vi "send_voltagePulse-v03.vi"(0 "daq_ao":tag="Dev1/ao1", 1 "daq_ai":tag="Dev1/ai0:1", 5 "VoltageRampValuesCluster":T2, 7 "Sample Freq (Hz)":dbl min=0.0 max=40000.0, 9 "set holding (mV)":dbl, 13 "Number of Replicates":i16=1 min=1 max=10, 14 "error in":errorcluster) -> (4 "output cluster":T1, 6 "output waveform":waveform(dbl)[](graph), 8 "protocol response":waveform(dbl)[](graph) caption="jumptestMonitor", 10 "error out":errorcluster)   [LabVIEW 2019]
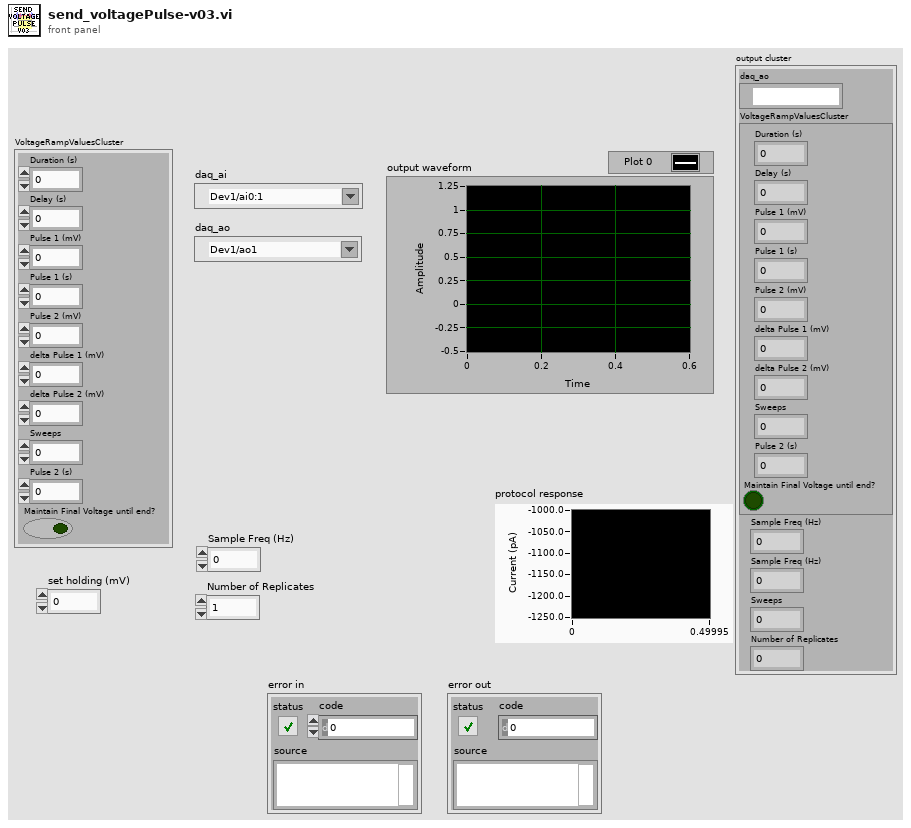
[diagram p1: front panel]
types:
  T1 = cluster{"daq_ao":tag, "VoltageRampValuesCluster":cluster{"Duration (s)":dbl, "Delay (s)":dbl, "Pulse 1 (mV)":dbl, "Pulse 1 (s)":dbl, "Pulse 2 (mV)":dbl, "delta Pulse 1 (mV)":dbl, "delta Pulse 2 (mV)":dbl, "Sweeps":dbl, "Pulse 2 (s)":dbl, "Maintain Final Voltage until end?":bool}, "Sample Freq (Hz)":dbl, "Sample Freq (Hz)":dbl, "Sweeps":dbl, "Number of Replicates":i16}
  T2 = cluster{"Duration (s)":dbl, "Delay (s)":dbl, "Pulse 1 (mV)":dbl, "Pulse 1 (s)":dbl, "Pulse 2 (mV)":dbl, "delta Pulse 1 (mV)":dbl, "delta Pulse 2 (mV)":dbl, "Sweeps":dbl, "Pulse 2 (s)":dbl, "Maintain Final Voltage until end?":bool}
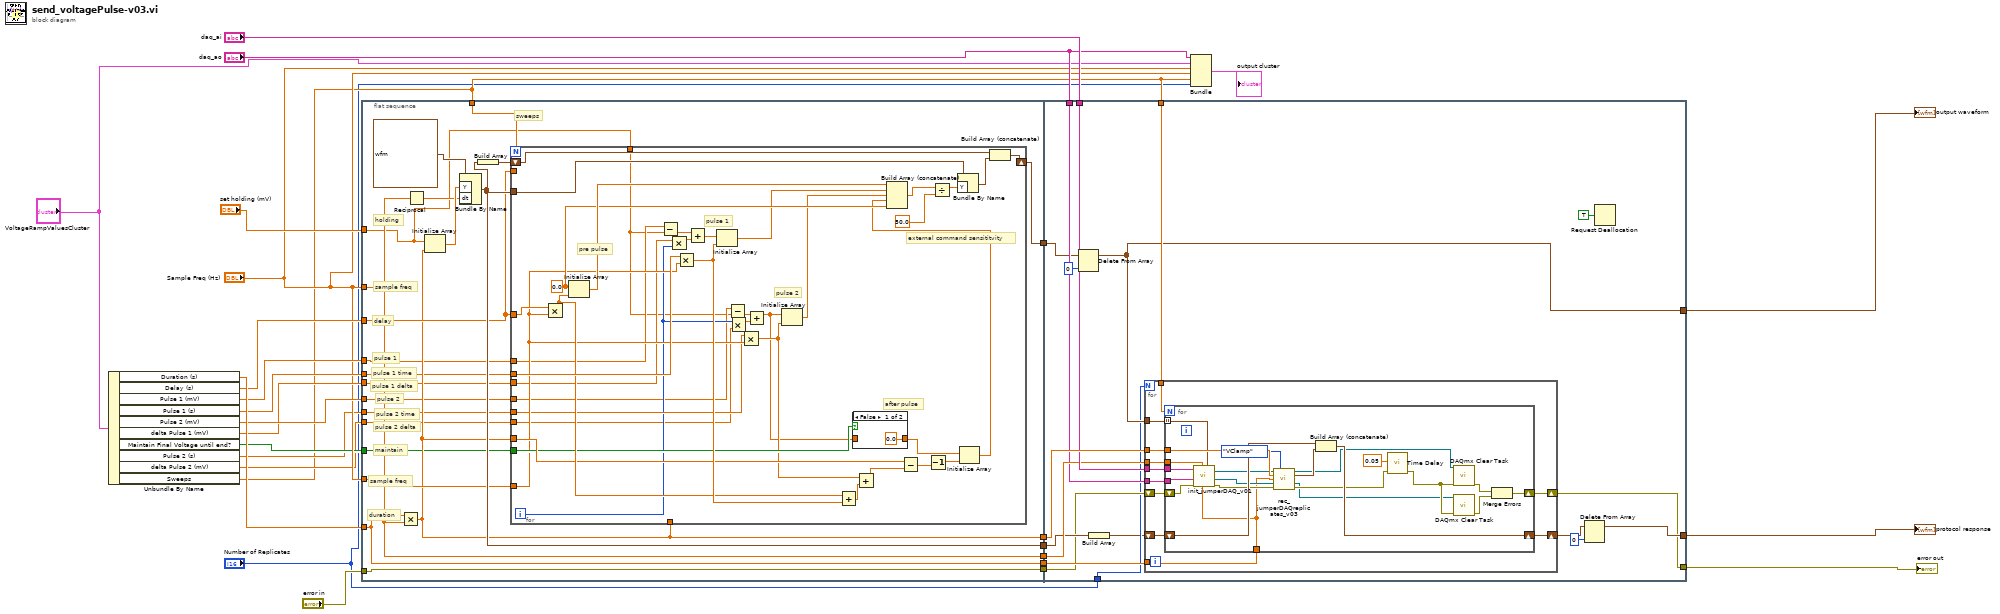
[diagram p0: block diagram]
diagram:
  n1 = Unbundle By Name("VoltageRampValuesCluster") -> ("Duration (s)"=w21:dbl, "Delay (s)"=w20:dbl, "Pulse 1 (mV)"=w19:dbl, "Pulse 1 (s)"=w11:dbl, "Pulse 2 (mV)"=w10:dbl, "delta Pulse 1 (mV)"=w9:dbl, "Maintain Final Voltage until end?"=w7:bool, "Pulse 2 (s)"=w4:dbl, "delta Pulse 2 (mV)"=w3:dbl, "Sweeps"=w2:dbl)
  n2 = flat-sequence {
    tunnel: w21 -> [w36]
    tunnel: "Sample Freq (Hz)" -> [w37]
    tunnel: [w35] -> w18
    tunnel: [w41] -> w17
    tunnel: [w42] -> w16
    tunnel: "error in" -> [w48]
    tunnel: [w48] -> w15
    tunnel: [w36] -> w14
    tunnel: w20 -> [w40]
    tunnel: w19 -> [w32]
    tunnel: [w47] -> w13
    tunnel: w2 -> [w46]
    tunnel: "Sample Freq (Hz)" -> [w41]
    tunnel: "set holding (mV)" -> [w38]
    tunnel: w11 -> [w31]
    tunnel: w10 -> [w30]
    tunnel: w9 -> [w34]
    tunnel: w7 -> [w33]
    tunnel: w4 -> [w29]
    tunnel: w3 -> [w28]
    tunnel: [w94] -> w27
    tunnel: w18 -> [w106]
    tunnel: "daq_ai" -> [w101]
    tunnel: "daq_ao" -> [w98]
    tunnel: w17 -> [w100]
    tunnel: [w104] -> w24
    tunnel: "Number of Replicates" -> [w91]
    tunnel: [w93] -> w22
    tunnel: w15 -> [w92]
    tunnel: w14 -> [w102]
    tunnel: w13 -> [w95]
    tunnel: w16 -> [w99]
    tunnel: w2 -> [w97]
    frame #0 {
      # "duration"
      # "sample freq"
      # "maintain"
      # "pulse 2 delta"
      # "pulse 2 time"
      # "pulse 2"
      # "pulse 1 delta"
      # "pulse 1 time"
      # "pulse 1"
      # "delay"
      # "sample freq"
      # "sweeps"
      # "holding"
      n3 = Multiply(x=w36, y=w41) -> (x*y=w35:dbl)
      n4 = Reciprocal(x=w41) -> (1/x=w39:dbl)
      n5 = Initialize Array(w38, w35) -> (w43:dbl[])
      n6 = Bundle By Name(cluster=waveform(dbl) {"t0"=timestamp(0 s since 1904-01-01), "dt"=1.0, "Y"=[]} ("signal out"), "Y"=w43, "dt"=w39) -> (w42:waveform(dbl))
      n7 = Build Array(w42) -> (w45:waveform(dbl)[])
      n8 = for {
        N: w46 -> [_]
        tunnel: w40 -> [_]
        shift-right: [w86] -> w47
        shift-left: w45 -> [w85]
        tunnel: w42 -> [w83]
        tunnel: w32 -> [w54]
        tunnel: w40 -> [w80]
        tunnel: w31 -> [w79]
        tunnel: w35 -> [_]
        tunnel: w38 -> [w51]
        tunnel: w37 -> [w67]
        tunnel: w34 -> [w60]
        tunnel: w35 -> [w73]
        tunnel: w33 -> [w69]
        tunnel: w30 -> [w52]
        tunnel: w29 -> [w66]
        tunnel: w28 -> [w56]
        i -> [w58]
        w78 = 0.0 ("element")
        # "external command sensititvity"
        # "after pulse"
        # "pulse 2"
        # "pulse 1"
        # "pre pulse"
        n9 = Multiply(x=w80, y=w67) -> (x*y=w74:dbl)
        n10 = Initialize Array(w78, w74) -> (w82:dbl[])
        n11 = Subtract(x=w54, y=w51) -> (x-y=w55:dbl)
        n12 = Multiply(x=w60, y=w58) -> (x*y=w61:dbl)
        n13 = Multiply(x=w79, y=w67) -> (x*y=w75:dbl)
        n14 = Add(x=w55, y=w61) -> (x+y=w62:dbl)
        n15 = Initialize Array(w62, w75) -> (w68:dbl[])
        n16 = Subtract(x=w52, y=w51) -> (x-y=w53:dbl)
        n17 = Multiply(x=w58, y=w56) -> (x*y=w57:dbl)
        n18 = Multiply(x=w66, y=w67) -> (x*y=w64:dbl)
        n19 = Add(x=w53, y=w57) -> (x+y=w59:dbl)
        n20 = Initialize Array(w59, w64) -> (w63:dbl[])
        n21 = Add(x=w74, y=w75) -> (x+y=w81:dbl)
        n22 = case shown="False" w69 {
          tunnel: w59 -> [_ w88]
          tunnel: [0.0 w88] -> w70
          frame False {
          }
          frame True {
          }
        }
        n23 = Add(x=w64, y=w81) -> (x+y=w65:dbl)
        n24 = Subtract(x=w73, y=w65) -> (x-y=w72:dbl)
        n25 = Decrement(x=w72) -> (x-1=w76:dbl)
        n26 = Initialize Array(w70, w76) -> (w77:dbl[])
        n27 = Build Array (concatenate)(w82, w68, w63, w77, w78) -> (w71:dbl[])
        n28 = Divide(x=w71, y=50.0) -> (x/y=w50:dbl[])
        n29 = Bundle By Name(cluster=w83, "Y"=w50) -> (w84:waveform(dbl))
        n30 = Build Array (concatenate)(w85, w84) -> (w86:waveform(dbl)[])
      }
    }
    frame #1 {
      n31 = Delete From Array(array=w95, index=0) -> (array with subset deleted=w94:waveform(dbl)[])  [unwired: 1 in, 1 out]
      n32 = Build Array(w99) -> (w90:waveform(dbl)[])
      n33 = for {
        N: w91 -> [_]
        tunnel: w106 -> [w117]
        tunnel: w102 -> [w115]
        tunnel: w101 -> [w114]
        tunnel: w100 -> [w113]
        tunnel: w98 -> [w112]
        tunnel: w97 -> [w111]
        tunnel: w94 -> [w110]
        shift-right: [w109] -> w93
        shift-left: w92 -> [w108]
        shift-right: [w116] -> w105
        shift-left: w90 -> [w107]
        n34 = for {
          N: w111 -> [_]
          tunnel: w117 -> [w139]
          shift-right: [w137] -> w116
          shift-left: w107 -> [w136]
          tunnel: w115 -> [w129]
          tunnel: w114 -> [w135]
          tunnel: w113 -> [w134]
          tunnel: w112 -> [w133]
          tunnel: w110 -> [w128] mode=indexing
          shift-right: [w123] -> w109
          shift-left: w108 -> [w122]
          n35 = call "init_jumperDAQ_v01.vi"("protocol waveform"=w128, "Duration (s)"=w129, "Sample Freq (Hz)"=w134, "AO error in"=w122, "AO physical channels"=w133, "AI Physical Channel"=w135) -> ("AO error out"=w132:errorcluster, "AO task out"=w131:refnum<k21>, "AI task out"=w130:refnum<k21>)  [unwired: 1 in, 2 out]
          n36 = call "rec_jumperDAQreplicates_v03.vi"("AI task in"=w130, "which clamp"=enum16{"VClamp", "IClamp"}."VClamp", "number of samples"=w139, "Duration (s)"=w129, "AO task in"=w131, "error in"=w132) -> ("AI task out"=w119:refnum<k21>, "data out (pA or mV)"=w138:waveform(dbl), "AO task out"=w120:refnum<k21>, "error out"=w126:errorcluster)  [unwired: 6 in]
          n37 = Build Array (concatenate)(w136, w138) -> (w137:waveform(dbl)[])
          n38 = call "Time Delay"("error in (no error)"=w126, "Delay Time (s)"=0.05) -> ("error out"=w121:errorcluster)  [unwired: 9 in]
          n39 = call <vilib>:"DAQmx Clear Task.vi"("task in"=w119, "error in"=w121) -> ("error out"=w125:errorcluster)  [unwired: 13 in]
          n40 = call <vilib>:"DAQmx Clear Task.vi"("task in"=w120, "error in"=w121) -> ("error out"=w124:errorcluster)  [unwired: 13 in]
          n41 = Merge Errors(w125, w124) -> (w123:errorcluster)
        }
      }
      n42 = Delete From Array(array=w105, index=0) -> (array with subset deleted=w104:waveform(dbl)[])  [unwired: 1 in, 1 out]
      n43 = Request Deallocation(TRUE ("flag")) -> ()
    }
  }
  n44 = Bundle("daq_ao"="daq_ao", "VoltageRampValuesCluster"="VoltageRampValuesCluster", "Sample Freq (Hz)"="Sample Freq (Hz)", "Sample Freq (Hz)"="Sample Freq (Hz)", "Sweeps"=w2, "Number of Replicates"="Number of Replicates") -> (→"output cluster":T1)  [unwired: 1 in]
  "protocol response" <- w24
  "output waveform" <- w27
  "error out" <- w22
